vi "Write Array Of WVFMs.vi"(8 "error in (no error)":errorcluster, 10 "Array":waveform(dbl)[](array[waveform]), 11 "RMS in":refnum<class "RMS.lvclass">) -> (0 "error out":errorcluster, 3 "RMS out":refnum<class "RMS.lvclass">)   [LabVIEW 2015, in "RMSLib.lvlib" / "RMS.lvclass"]
uses:
  RMS.lvclass
  RMS.lvclass/RMS.ctl
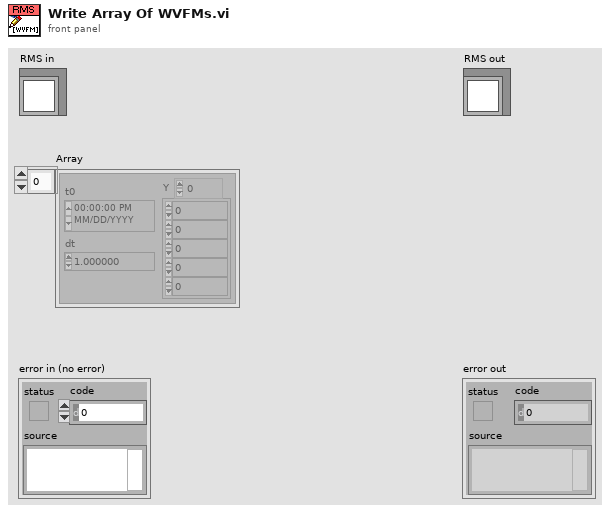
[diagram p1: front panel]
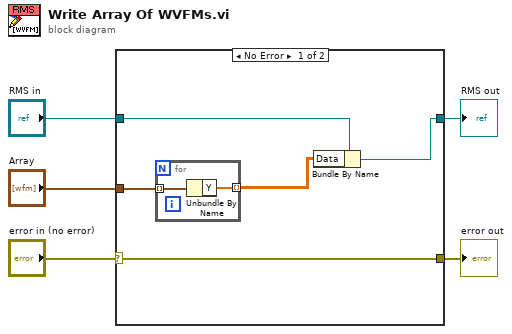
[diagram p0: block diagram]
diagram:
  n1 = case shown="No Error" "error in (no error)" {
    selector: "error in (no error)" -> [w8 w14]
    tunnel: [w8 w14] -> w4
    tunnel: "RMS in" -> [w10 w13]
    tunnel: [w9 w13] -> w2
    tunnel: "Array" -> [w7 _]
    frame No Error {
      n2 = for {
        tunnel: w7 -> [w12] mode=indexing
        tunnel: [w11] -> w6 mode=indexing
        n3 = Unbundle By Name(w12) -> ("Y"=w11:dbl[])
      }
      n4 = Bundle By Name(cluster=w10, "Data"=w6) -> (w9:refnum<class "RMS.lvclass">)
    }
    frame Error {
    }
  }
  "error out" <- w4
  "RMS out" <- w2
